vi "PXI6251_ai.vi"() -> ()   [LabVIEW 2017]
doc: "Use this template to build a producer/consumer design pattern with events to produce queue items. Use this design pattern instead of the User Interface Event Handler pattern for user interfaces when you want to execute code asynchronously in response to an event without slowing the user interface responsiveness."
uses:
  controls/QI_6251ai.ctl
  controls/FS_PXI6521ai.ctl
  Hardware/PXI6251_AI/Command.ctl
  UIchange/GuideTree/FGV_GuideTree.ctl
panel:
  in  "Save?":bool
  in  "文件路径":path
  in  "Start/Stop":bool
  in  "采样速率":dbl=10000.0
  out "Waveform Graph":waveform(dbl)[](graph)=[{"t0"=timestamp(0 s since 1904-01-01), "dt"=1.0, "Y"=[], "attributes"=variant("NI_ChannelName"=variant(string "Dev01/ai0"), "NI_UnitDescription"=variant(string "Volts"))}, {"t0"=timestamp(0 s since 1904-01-01), "dt"=1.0, "Y"=[], "attributes"=variant("NI_ChannelName"=variant(string "Dev01/ai2"), "NI_UnitDescription"=variant(string "Volts"))}]
  in  "模式":i32(slide) scale=0.0..1.0
  in  "Sing_ch":T1
  in  "Diff_ch":T2={"ai00"=TRUE, "ai01"=FALSE, "ai02"=TRUE, "ai03"=FALSE, "ai04"=FALSE, "ai05"=FALSE, "ai06"=FALSE, "ai07"=FALSE}
  # "PXI-6251模拟信号采集器"
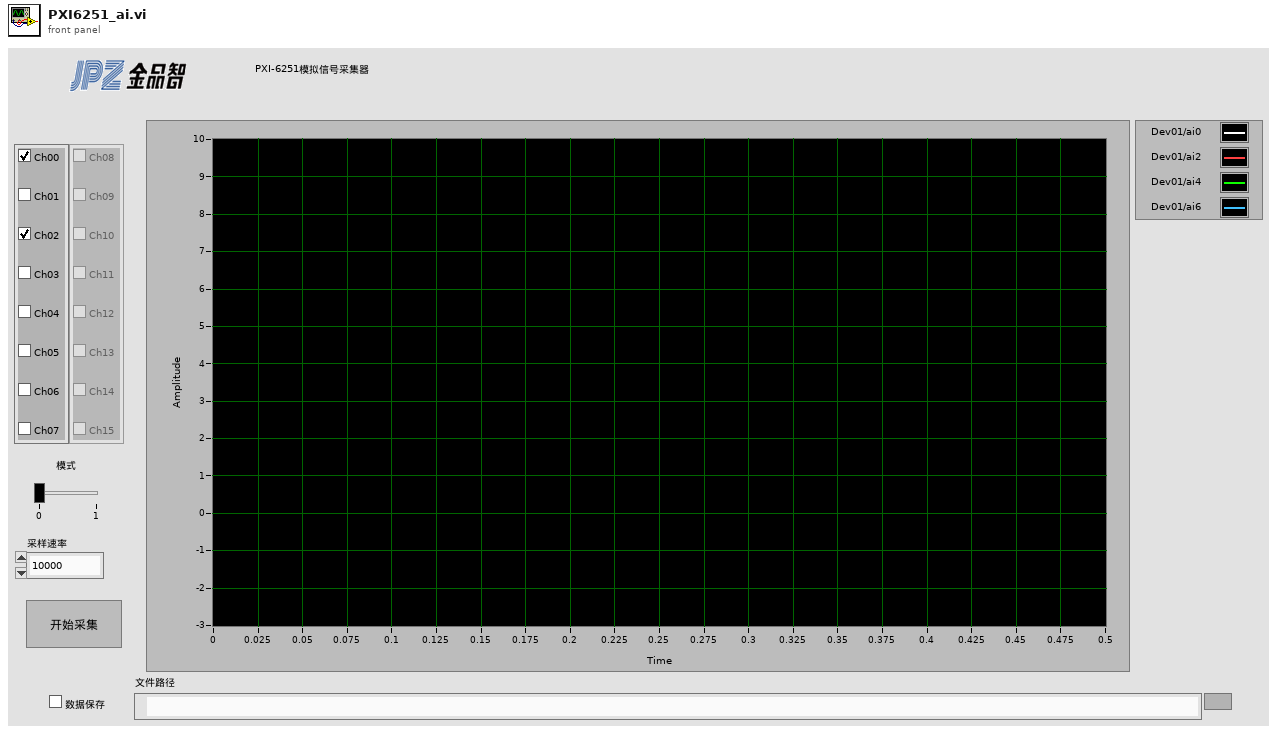
[diagram p1: front panel]
types:
  T1 = cluster{"ai08":bool, "ai09":bool, "ai10":bool, "ai11":bool, "ai12":bool, "ai13":bool, "ai14":bool, "ai15":bool}
  T2 = cluster{"ai00":bool, "ai01":bool, "ai02":bool, "ai03":bool, "ai04":bool, "ai05":bool, "ai06":bool, "ai07":bool}
  T3 = typedef "QI_6251ai.ctl" = cluster{"State":T4, "data":variant}
  T4 = typedef "FS_PXI6521ai.ctl" = enum16{"Initialize", "Mode chang", "idel", "Start acquire", "Read data", "Stop acquire"}
  T5 = typedef "Command.ctl" = enum16{"Start Acquire", "Read Data", "Release task"}
  T6 = typedef "FGV_GuideTree.ctl" = enum16{"SetTree*", "GetTree*", "InitlizeTree", "Get Item infor"}
  T7 = cluster{"Channel":string[], "Sample rate":dbl, "input terminal configuration":i32}
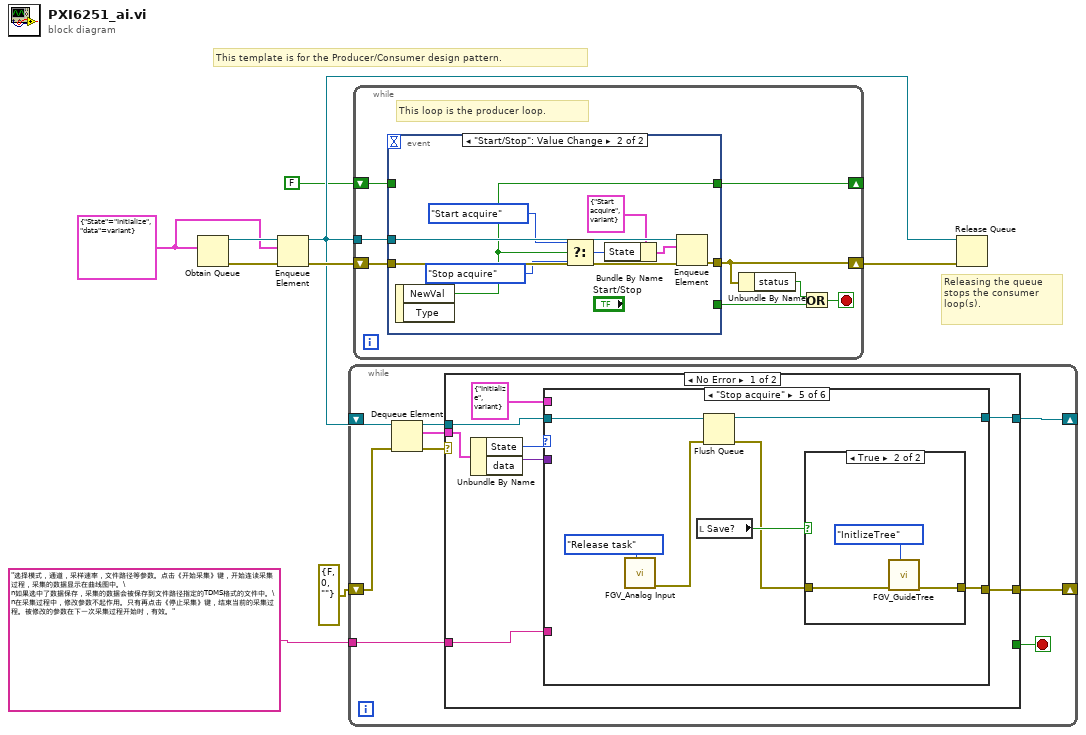
[diagram p0: block diagram]
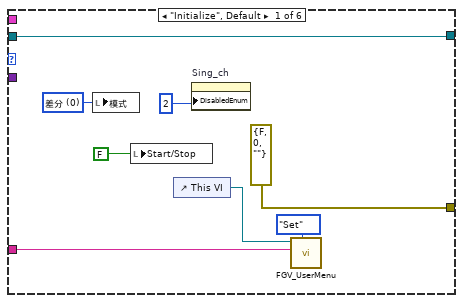
[diagram p2: hidden frame]
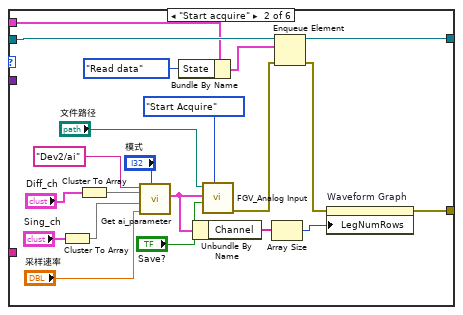
[diagram p3: hidden frame]
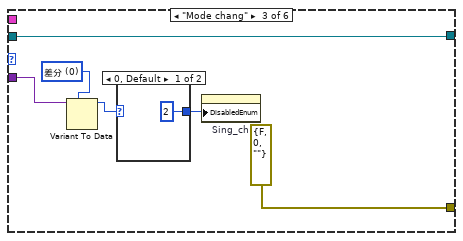
[diagram p4: hidden frame]
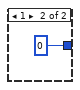
[diagram p5: hidden frame]
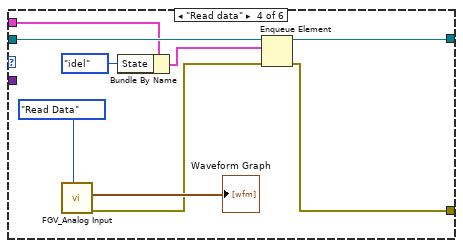
[diagram p6: hidden frame]
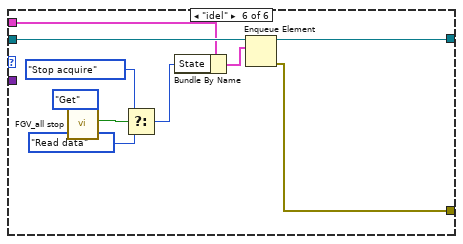
[diagram p8: hidden frame]
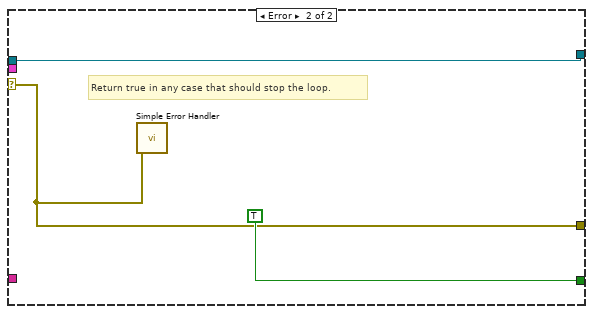
[diagram p9: hidden frame]
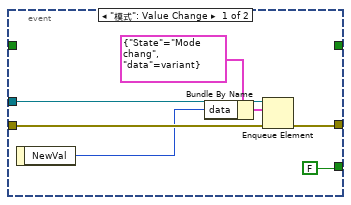
[diagram p10: hidden frame]
diagram:
  w4 = T3 {"State"=enum."Initialize", "data"=variant(string "")}
  # "Releasing the queue stops the consumer loop(s)."
  # "This template is for the Producer/Consumer design pattern."
  n1 = Obtain Queue(element data type=w4) -> (queue out=w6:refnum<queue>, error out=w8:errorcluster)  [unwired: 4 in, 1 out]
  n2 = Enqueue Element(queue=w6, element=w4) -> (queue out=w5:refnum<queue>)  [unwired: 2 in, 2 out]
  n3 = while {
    shift-right: [w13] -> _
    shift-left: errorcluster {"status"=FALSE, "code"=0, "source"=""} ("error IO") -> [w12]
    shift-right: [w10] -> _
    shift-left: w5 -> [w17]
    tunnel: "选择模式，通道，采样速率，文件路径等参数。点击《开始采集》键，开始连读采集过程，采集的数据显示在曲线图中。\n如果选中了数据保存，采集的数据会被保存到文件路径指定的TDMS格式的文件中。\n在采集过程中，修改参数不起作用。只有再点击《停止采集》键，结束当前的采集过程。被修改的参数在下一次采集过程开始时，有效。" -> [w9]
    stop <- w14 stop-if-true
    n4 = Dequeue Element(queue=w17, error in (no error)=w12) -> (queue out=w11:refnum<queue>, element=w15:T3, error out=w16:errorcluster)  [unwired: 1 in, 1 out]
    n5 = case shown="No Error" w16 {
      selector: w16 -> [_ w93]
      tunnel: w15 -> [w25 _]
      tunnel: [_ TRUE] -> w14
      tunnel: [w22 w93] -> w13
      tunnel: w11 -> [w21 w94]
      tunnel: [w20 w94] -> w10
      tunnel: w9 -> [w18 _]
      frame No Error {
        n6 = Unbundle By Name(w25) -> ("State"=w24:T4, "data"=w23:variant)
        n7 = case shown="\"Stop acquire\"" w24 {
          tunnel: w23 -> [_ _ w60 _ _ _]
          tunnel: [errorcluster {"status"=FALSE, "code"=0, "source"=""} ("error out") w35 errorcluster {"status"=FALSE, "code"=0, "source"=""} ("error out") w66 w72 w89] -> w22
          tunnel: w21 -> [w30 w52 w55 w69 w75 w91]
          tunnel: [w30 w50 w55 w68 w76 w90] -> w20
          tunnel: T3 {"State"=enum."Initialize", "data"=variant(string "")} -> [_ w49 _ w65 _ w88]
          tunnel: w18 -> [w26 _ _ _ _ _]
          frame "Initialize", Default {
            w33 = 0 items=["差分", "单端"] ("模式")
            n8 = local write "模式"(w33) -> ()
            n9 = local write "Start/Stop"(FALSE) -> ()
            n10 = control-ref of="This VI"() -> (w27:refnum<vi>)
            n11 = property on="Sing_ch" class="Clust (strict)"("DisabledEnum"=2) -> ()  [unwired: 2 in, 2 out]
            n12 = call "FGV_UserMenu.vi"("Command"=enum16{"Initialize", "Set", "Get"}."Set", "Use Info"=w26, "VI Refnum"=w27) -> ()  [unwired: 8 in, 1 out]
          }
          frame "Start acquire" {
            n13 = Cluster To Array(cluster="Sing_ch") -> (array=w42:bool[])
            n14 = Cluster To Array(cluster="Diff_ch") -> (array=w40:bool[])
            n15 = call "Get ai_parameter.vi"("模式"="模式", "采样速率"="采样速率", "Sing_ch"=w42, "Diff_ch"=w40, "Device name"="Dev2/ai") -> ("Daq_ai_para"=w38:T7)  [unwired: 6 in]
            n16 = Bundle By Name(cluster=w49, "State"=FS_PXI6521ai."Read data") -> (w48:T3)
            n17 = Unbundle By Name(w38) -> ("Channel"=w37:string[])
            n18 = call "FGV_Analog Input.vi"("Command"=Command."Start Acquire", "Save data?"="Save?", "Daq_ai_para"=w38, "TDMS File Path"="文件路径") -> ("error out"=w51:errorcluster)  [unwired: 5 in, 2 out]
            n19 = Array Size(array=w37) -> (size(s)=w34:i32)
            n20 = Enqueue Element(queue=w52, element=w48, error in (no error)=w51) -> (queue out=w50:refnum<queue>, error out=w36:errorcluster)  [unwired: 1 in, 1 out]
            n21 = property on="Waveform Graph" class="WFGraph (strict)"(error in=w36, "LegNumRows"=w34) -> (error out=w35:errorcluster)  [unwired: 1 in, 1 out]
          }
          frame "Mode chang" {
            w59 = 0 items=["差分", "单端"] ("模式")
            n22 = Variant To Data(type=w59, Variant=w60) -> (data=w58:i32)  [unwired: 1 in, 1 out]
            n23 = case shown="0, Default" w58 {
              tunnel: [2 0] -> w57
              frame 0, Default {
              }
              frame 1 {
              }
            }
            n24 = property on="Sing_ch" class="Clust (strict)"("DisabledEnum"=w57) -> ()  [unwired: 2 in, 2 out]
          }
          frame "Read data" {
            n25 = call "FGV_Analog Input.vi"("Command"=Command."Read Data") -> ("error out"=w67:errorcluster, "data"=→"Waveform Graph":waveform(dbl)[])  [unwired: 8 in, 1 out]
            n26 = Bundle By Name(cluster=w65, "State"=FS_PXI6521ai."idel") -> (w63:T3)
            n27 = Enqueue Element(queue=w69, element=w63, error in (no error)=w67) -> (queue out=w68:refnum<queue>, error out=w66:errorcluster)  [unwired: 1 in, 1 out]
          }
          frame "Stop acquire" {
            n28 = call "FGV_Analog Input.vi"("Command"=Command."Release task") -> ("error out"=w77:errorcluster)  [unwired: 8 in, 2 out]
            n29 = local read "Save?"() -> (w74:bool)
            n30 = Flush Queue(queue=w75, error in (no error)=w77) -> (queue out=w76:refnum<queue>, error out=w73:errorcluster)  [unwired: 1 out]
            n31 = case shown="True" w74 {
              tunnel: w73 -> [w79 w82]
              tunnel: [w79 w81] -> w72
              frame False {
              }
              frame True {
                n32 = call "FGV_GuideTree.vi"("Action"=FGV_GuideTree."InitlizeTree", "error in"=w82) -> ("error out"=w81:errorcluster)  [unwired: 6 in, 3 out]
              }
            }
          }
          frame "idel" {
            n33 = call "FGV_all stop.vi"("Enum"=enum16{"Set", "Get"}."Get") -> ("All Stop?"=w86:bool)  [unwired: 10 in]
            n34 = Select(t=FS_PXI6521ai."Stop acquire" ("State"), s=w86, f=FS_PXI6521ai."Read data" ("State")) -> (s? t:f=w84:T4)
            n35 = Bundle By Name(cluster=w88, "State"=w84) -> (w87:T3)
            n36 = Enqueue Element(queue=w91, element=w87) -> (queue out=w90:refnum<queue>, error out=w89:errorcluster)  [unwired: 2 in, 1 out]
          }
        }
      }
      frame Error {
        # "Return true in any case that should stop the loop."
        n37 = call <vilib>:"Simple Error Handler.vi"("error in (no error)"=w93) -> ()  [unwired: 4 in, 5 out]
      }
    }
  }
  n38 = while {
    shift-right: [w99] -> w7
    shift-left: w8 -> [w102]
    tunnel: w5 -> [w103]
    shift-right: [w96] -> _
    shift-left: FALSE -> [w97]
    stop <- w100 stop-if-true
    # "This loop is the producer loop."
    n39 = event shown="[1] \"Start/Stop\": Value Change" {
      selector: _ -> [_ _]
      dyn-events: _ -> [_ _]
      timeout: _ -> [_ _]
      tunnel: w103 -> [w109 w117]
      tunnel: w102 -> [w110 w119]
      tunnel: [w108 w118] -> w99
      tunnel: [FALSE _] -> w101
      tunnel: w97 -> [_ _]
      tunnel: [_ w111] -> w96
      event "模式": Value Change {
        n40 = event-data() -> ("NewVal"=w105:i32)  [unwired: 1 in]
        n41 = Bundle By Name(cluster=T3 {"State"=enum."Mode chang", "data"=variant} ("element"), "data"=w105) -> (w106:T3)
        n42 = Enqueue Element(queue=w109, element=w106, error in (no error)=w110) -> (error out=w108:errorcluster)  [unwired: 1 in, 2 out]
      }
      event "Start/Stop": Value Change {
        n43 = event-data() -> ("NewVal"=w111:bool)  [unwired: 1 in, 1 out]
        n44 = Select(t=FS_PXI6521ai."Start acquire" ("State"), s=w111, f=FS_PXI6521ai."Stop acquire" ("State")) -> (s? t:f=w112:T4)
        n45 = Bundle By Name(cluster=T3 {"State"=enum."Start acquire", "data"=variant} ("element"), "State"=w112) -> (w115:T3)
        n46 = Enqueue Element(queue=w117, element=w115, error in (no error)=w119) -> (error out=w118:errorcluster)  [unwired: 1 in, 2 out]
      }
    }
    n47 = Unbundle By Name(w99) -> ("status"=w98:bool)
    n48 = Or(x=w98, y=w101) -> (x .or. y?=w100:bool)
  }
  n49 = Release Queue(queue=w5, error in (no error)=w7) -> ()  [unwired: 1 in, 3 out]
